vi "TOPAZ.vi"() -> ()   [LabVIEW 2018]
uses:
  <vilib>/Instr/_visa.llb/VISA Configure Serial Port (Instr).vi
panel:
  in  "stop":bool
  in  "COM - порт":refnum<visa-resource-name>="COM14"
  in  "Доступные длины\nволн? (нм)":bool
  in  "Установить":bool
  in  "Установить":bool
  in  "Ослабление, дБ":string
  in  "Длина волны, нм":string
  in  "Текущее ослабление? (дБ)":bool
  in  "Текущая длина\nволны? (нм)":bool
  out "Ответ:":string
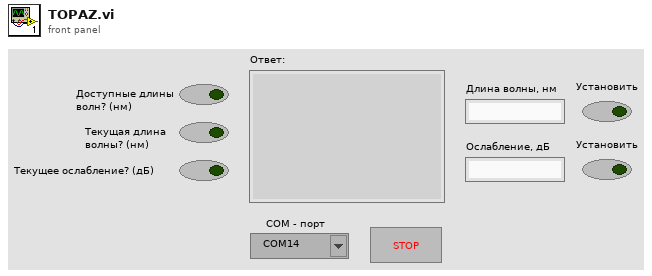
[diagram p1: front panel]
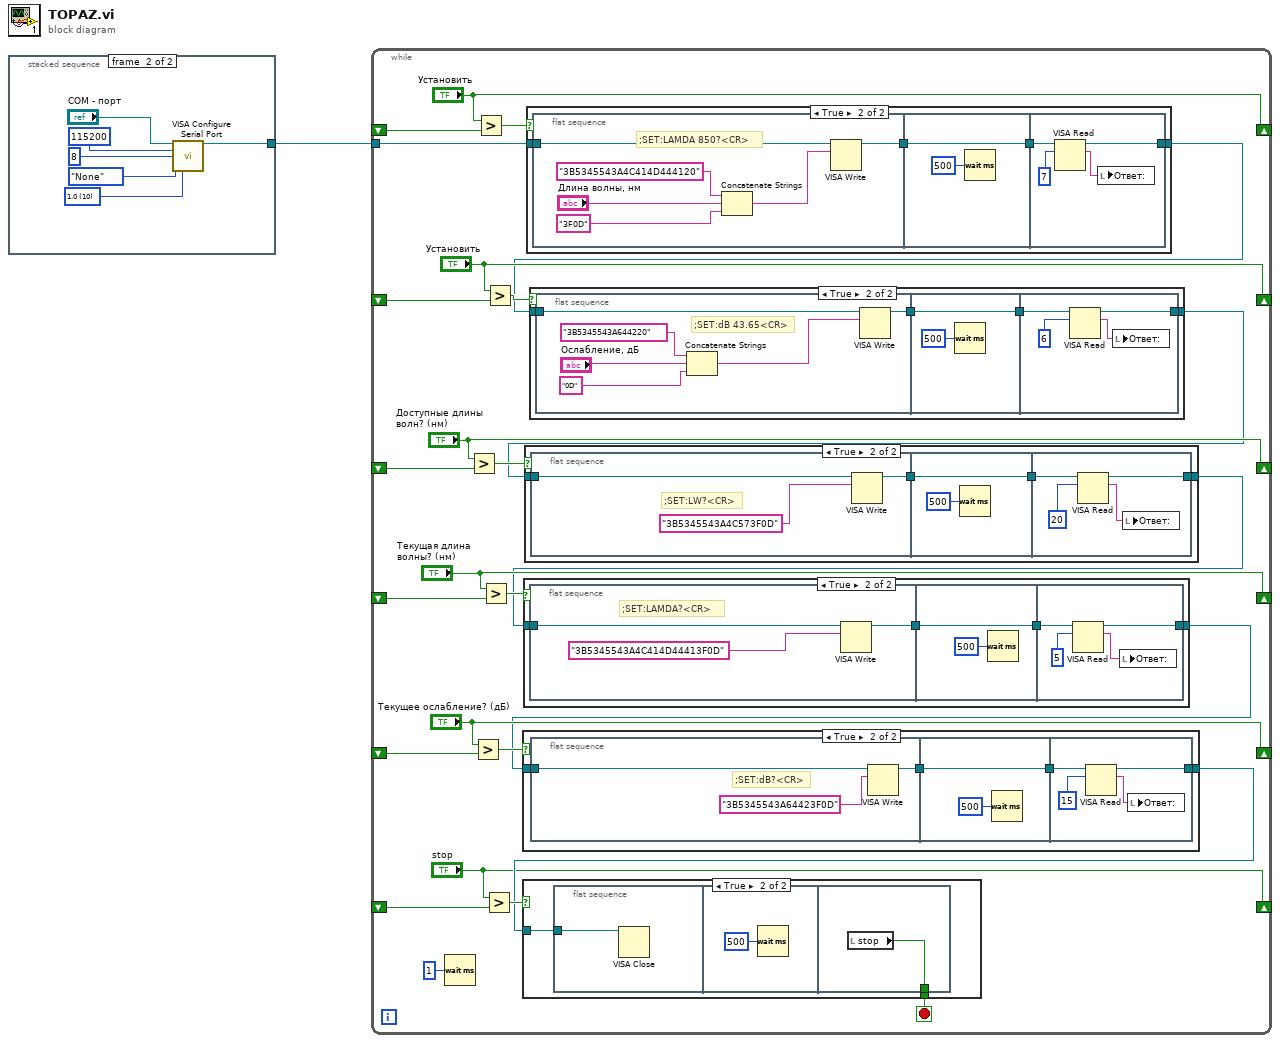
[diagram p0: block diagram]
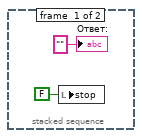
[diagram p2: hidden frame]
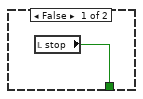
[diagram p3: hidden frame]
diagram:
  n1 = stacked-sequence {
    tunnel: [_ w4] -> w1
    frame #0 {
      n2 = local write "stop"(FALSE ("stop")) -> ()
      "Ответ:" <- "" ("Ответ:")
    }
    frame #1 {
      w6 = u16 10 items=["1.0"=10, "1.5"=15, "2.0"=20] ("stop bits (10: 1 bit)")
      n3 = call-poly "VISA Configure Serial Port"("VISA resource name"="COM - порт", "baud rate (9600)"=u32 115200, "data bits (8)"=u16 8, "parity (0:none)"=enum16{"None", "Odd", "Even", "Mark", "Space"}."None", "stop bits (10: 1 bit)"=w6) -> ("VISA resource name out"=w4:refnum<visa-resource-name>)  [unwired: 9 in, 1 out]
    }
  }
  n4 = while {
    shift-right: ["Установить"] -> _
    shift-left: _ -> [w35]
    tunnel: w1 -> [w31]
    shift-right: ["Установить"] -> _
    shift-left: _ -> [w30]
    shift-right: ["Доступные длины\nволн? (нм)"] -> _
    shift-left: _ -> [w23]
    shift-right: ["Текущая длина\nволны? (нм)"] -> _
    shift-left: _ -> [w20]
    shift-right: ["Текущее ослабление? (дБ)"] -> _
    shift-left: _ -> [w18]
    shift-right: ["stop"] -> _
    shift-left: _ -> [w14]
    stop <- w10 stop-if-true
    n5 = Wait (ms)(milliseconds to wait=u32 1) -> ()  [unwired: 1 out]
    n6 = Greater?(x="Доступные длины\nволн? (нм)", y=w23) -> (0:w25:bool)
    n7 = Greater?(x="Текущее ослабление? (дБ)", y=w18) -> (0:w16:bool)
    n8 = Greater?(x="Установить", y=w35) -> (0:w33:bool)
    n9 = Greater?(x="Текущая длина\nволны? (нм)", y=w20) -> (0:w22:bool)
    n10 = Greater?(x="stop", y=w14) -> (0:w13:bool)
    n11 = Greater?(x="Установить", y=w30) -> (0:w28:bool)
    n12 = case shown="True" w33 {
      tunnel: w31 -> [w101 w105]
      tunnel: [w101 w102] -> w27
      frame False {
      }
      frame True {
        n13 = flat-sequence {
          tunnel: w105 -> [w111]
          tunnel: [w110] -> w103
          tunnel: [w112] -> w104
          tunnel: w103 -> [w112]
          tunnel: w104 -> [w117]
          tunnel: [w115] -> w102
          frame #0 {
            # ";SET:LAMDA 850?<CR>"
            n14 = Concatenate Strings("3B5345543A4C414D444120", "Длина волны, нм", "3F0D") -> (w106:string)
            n15 = VISA Write(VISA resource name=w111, write buffer=w106) -> (VISA resource name out=w110:refnum<visa-resource-name>)  [unwired: 1 in, 2 out]
          }
          frame #1 {
            n16 = Wait (ms)(milliseconds to wait=u32 500) -> ()  [unwired: 1 out]
          }
          frame #2 {
            n17 = VISA Read(VISA resource name=w117, byte count=u32 7) -> (VISA resource name out=w115:refnum<visa-resource-name>, read buffer=w116:string)  [unwired: 1 in, 2 out]
            n18 = local write "Ответ:"(w116) -> ()
          }
        }
      }
    }
    n19 = case shown="True" w28 {
      tunnel: w27 -> [w84 w88]
      tunnel: [w84 w85] -> w24
      frame False {
      }
      frame True {
        n20 = flat-sequence {
          tunnel: w88 -> [w94]
          tunnel: [w93] -> w87
          tunnel: w87 -> [w96]
          tunnel: [w96] -> w86
          tunnel: w86 -> [w100]
          tunnel: [w98] -> w85
          frame #0 {
            # ";SET:dB 43.65<CR>"
            n21 = Concatenate Strings("3B5345543A644220", "Ослабление, дБ", "0D") -> (w89:string)
            n22 = VISA Write(VISA resource name=w94, write buffer=w89) -> (VISA resource name out=w93:refnum<visa-resource-name>)  [unwired: 1 in, 2 out]
          }
          frame #1 {
            n23 = Wait (ms)(milliseconds to wait=u32 500) -> ()  [unwired: 1 out]
          }
          frame #2 {
            n24 = VISA Read(VISA resource name=w100, byte count=u32 6) -> (VISA resource name out=w98:refnum<visa-resource-name>, read buffer=w99:string)  [unwired: 1 in, 2 out]
            n25 = local write "Ответ:"(w99) -> ()
          }
        }
      }
    }
    n26 = case shown="True" w25 {
      tunnel: w24 -> [w70 w74]
      tunnel: [w70 w71] -> w19
      frame False {
      }
      frame True {
        n27 = flat-sequence {
          tunnel: w74 -> [w77]
          tunnel: [w76] -> w72
          tunnel: [w78] -> w73
          tunnel: w72 -> [w78]
          tunnel: w73 -> [w83]
          tunnel: [w82] -> w71
          frame #0 {
            # ";SET:LW?<CR>"
            n28 = VISA Write(VISA resource name=w77, write buffer="3B5345543A4C573F0D") -> (VISA resource name out=w76:refnum<visa-resource-name>)  [unwired: 1 in, 2 out]
          }
          frame #1 {
            n29 = Wait (ms)(milliseconds to wait=u32 500) -> ()  [unwired: 1 out]
          }
          frame #2 {
            n30 = VISA Read(VISA resource name=w83, byte count=u32 20) -> (VISA resource name out=w82:refnum<visa-resource-name>, read buffer=w81:string)  [unwired: 1 in, 2 out]
            n31 = local write "Ответ:"(w81) -> ()
          }
        }
      }
    }
    n32 = case shown="True" w22 {
      tunnel: w19 -> [w56 w60]
      tunnel: [w56 w57] -> w15
      frame False {
      }
      frame True {
        n33 = flat-sequence {
          tunnel: w60 -> [w63]
          tunnel: [w62] -> w58
          tunnel: [w64] -> w59
          tunnel: w58 -> [w64]
          tunnel: w59 -> [w68]
          tunnel: [w67] -> w57
          frame #0 {
            # ";SET:LAMDA?<CR>"
            n34 = VISA Write(VISA resource name=w63, write buffer="3B5345543A4C414D44413F0D") -> (VISA resource name out=w62:refnum<visa-resource-name>)  [unwired: 1 in, 2 out]
          }
          frame #1 {
            n35 = Wait (ms)(milliseconds to wait=u32 500) -> ()  [unwired: 1 out]
          }
          frame #2 {
            n36 = VISA Read(VISA resource name=w68, byte count=u32 5) -> (VISA resource name out=w67:refnum<visa-resource-name>, read buffer=w69:string)  [unwired: 1 in, 2 out]
            n37 = local write "Ответ:"(w69) -> ()
          }
        }
      }
    }
    n38 = case shown="True" w16 {
      tunnel: w15 -> [w42 w46]
      tunnel: [w42 w43] -> w12
      frame False {
      }
      frame True {
        n39 = flat-sequence {
          tunnel: w46 -> [w49]
          tunnel: [w48] -> w44
          tunnel: [w50] -> w45
          tunnel: w44 -> [w50]
          tunnel: w45 -> [w54]
          tunnel: [w53] -> w43
          frame #0 {
            # ";SET:dB?<CR>"
            n40 = VISA Write(VISA resource name=w49, write buffer="3B5345543A64423F0D") -> (VISA resource name out=w48:refnum<visa-resource-name>)  [unwired: 1 in, 2 out]
          }
          frame #1 {
            n41 = Wait (ms)(milliseconds to wait=u32 500) -> ()  [unwired: 1 out]
          }
          frame #2 {
            n42 = VISA Read(VISA resource name=w54, byte count=u32 15) -> (VISA resource name out=w53:refnum<visa-resource-name>, read buffer=w55:string)  [unwired: 1 in, 2 out]
            n43 = local write "Ответ:"(w55) -> ()
          }
        }
      }
    }
    n44 = case shown="True" w13 {
      tunnel: w12 -> [_ w38]
      tunnel: [w36 w37] -> w10
      frame False {
        n45 = local read "stop"() -> (w36:bool)
      }
      frame True {
        n46 = flat-sequence {
          tunnel: w38 -> [w39]
          tunnel: [w41] -> w37
          frame #0 {
            n47 = VISA Close(VISA resource name=w39) -> ()  [unwired: 1 in, 1 out]
          }
          frame #1 {
            n48 = Wait (ms)(milliseconds to wait=u32 500) -> ()  [unwired: 1 out]
          }
          frame #2 {
            n49 = local read "stop"() -> (w41:bool)
          }
        }
      }
    }
  }
